vi "Check Log Status.vi"(8 "error in":errorcluster, 11 "PCAP Frame Logger in":refnum<class "PCAP Frame Logger.lvclass">) -> (0 "error out":errorcluster, 2 "Log file Size MB":dbl, 3 "PCAP Frame Logger out":refnum<class "PCAP Frame Logger.lvclass">, 4 "Hard Drive Space Used (%)":dbl, 5 "current filename":path)   [LabVIEW 2020, in "Frame Logging.lvlib" / "PCAP Frame Logger.lvclass"]
uses:
  PCAP Frame Logger.lvclass
  <resource>/objmgr/nisysapi.rc
  <vilib>/Utility/SystemLogging/NI_SystemLogging.lvlib
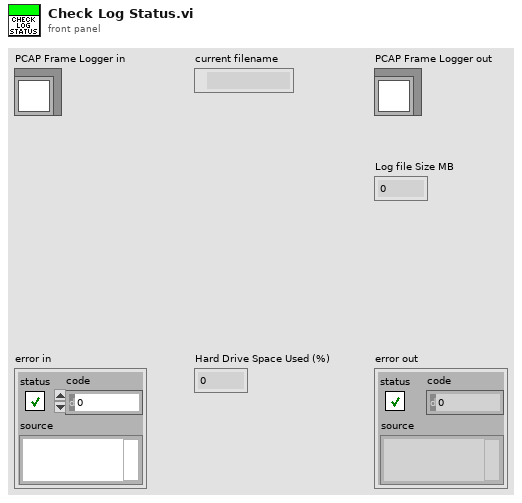
[diagram p1: front panel]
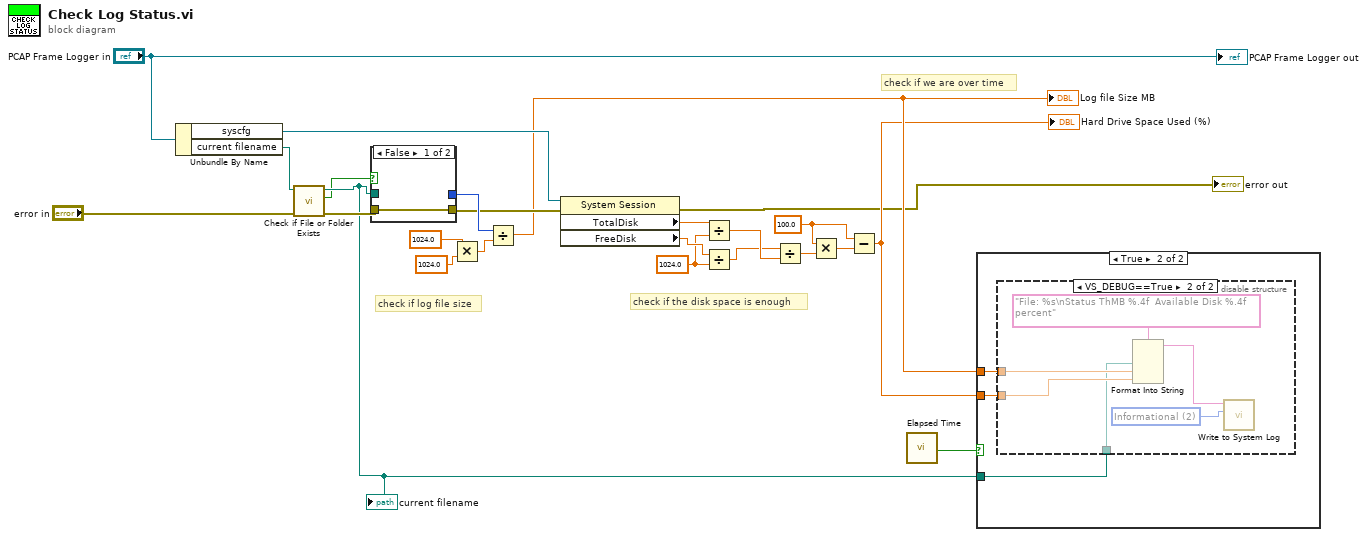
[diagram p0: block diagram]
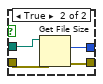
[diagram p2: hidden frame]
diagram:
  w19 = 100.0 ("y")
  w21 = 1024.0
  # "check if log file size"
  # "check if we are over time"
  # "check if the disk space is enough"
  n1 = Unbundle By Name("PCAP Frame Logger in") -> ("syscfg"=w15:refnum<k21>, "current filename"=w4:path)
  n2 = call <vilib>:"Check if File or Folder Exists.vi"("error in (no error)"="error in", "path"=w4) -> ("error out"=w3:errorcluster, "file or folder exists?"=w1:bool, "dup path"=w2:path)  [unwired: 7 in]
  "current filename" <- w2
  n3 = case shown="False" w1 {
    tunnel: [_ w29] -> w14
    tunnel: [w25 w28] -> w10
    tunnel: w3 -> [w25 w27]
    tunnel: w2 -> [_ w26]
    frame False {
    }
    frame True {
      n4 = Get File Size(file=w26, error in=w27) -> (size (in bytes)=w29:i64, 0:w28:errorcluster)  [unwired: 1 out]
    }
  }
  n5 = Multiply(x=1024.0, y=1024.0) -> (x*y=w11:dbl)
  n6 = Divide(x=w14, y=w11) -> (x/y=w9:dbl)
  "Log file Size MB" <- w9
  n7 = property class="System Session"(reference=w15, error in=w10) -> (error out=→"error out":errorcluster, "TotalDisk"=w23:dbl, "FreeDisk"=w22:dbl)  [unwired: 1 out]
  n8 = Divide(x=w23, y=w21) -> (x/y=w17:dbl)
  n9 = Divide(x=w22, y=w21) -> (x/y=w16:dbl)
  n10 = Divide(x=w16, y=w17) -> (x/y=w20:dbl)
  n11 = Multiply(x=w19, y=w20) -> (x*y=w18:dbl)
  n12 = Subtract(x=w19, y=w18) -> (x-y=w8:dbl)
  "Hard Drive Space Used (%)" <- w8
  n13 = call "Elapsed Time"() -> ("Time has Elapsed"=w7:bool)  [unwired: 12 in, 7 out]
  n14 = case shown="True" w7 {
    tunnel: w9 -> [_ w32]
    tunnel: w8 -> [_ w31]
    tunnel: w2 -> [_ w30]
    frame False {
    }
    frame True {
      n15 = disable-structure shown="VS_DEBUG==True" {
        disable-tunnel: w32 -> [_ w35]
        disable-tunnel: w31 -> [_ w34]
        disable-tunnel: w30 -> [_ w33]
        frame condition #0 (active) {
        }
        frame condition #1 {
          w36 = 2 items=["Error", "Warning", "Informational"] ("severity")
          n16 = Format Into String(format string="File: %s\nStatus ThMB %.4f  Available Disk %.4f percent", w33, w35, w34) -> (resulting string=w37:string)  [unwired: 2 in, 1 out]
          n17 = call <vilib>:"Write to System Log.vi"("severity"=w36, "message"=w37) -> ()  [unwired: 9 in, 1 out]
        }
      }
    }
  }
  "PCAP Frame Logger out" <- "PCAP Frame Logger in"
